vi "Main.vi"(8 "error in":errorcluster, 11 "Aging View in":refnum<class "Aging View.lvclass">) -> (0 "error out":errorcluster, 3 "Aging View out":refnum<class "Aging View.lvclass">)   [LabVIEW 2018, in "Aging View.lvclass"]
doc: "The Queued Message Handler of a Worker."
uses:
  Aging View.lvclass
  D:/Program Files (x86)/National Instruments/LabVIEW 2018/vi.lib/addons/_Workers/Library/Classes/Worker/Worker.lvclass
  Slot.ctl
  Initialization Data.ctl
  <vilib>/addons/_Workers/Library/Classes/Message Queue/Message Queue.lvclass
  Aging View.lvclass/Aging View.ctl
  <vilib>/addons/_Workers/Library/Classes/Message/Priority.ctl
  Datas.ctl
  <vilib>/addons/_Workers/Library/Classes/Message/Enqueue Message to Queue.vi
  <vilib>/addons/_Workers/Library/Classes/Message/Enqueue Message to Self v2.vi
  <vilib>/addons/_Workers/Library/Classes/Worker/Worker.lvclass
  <vilib>/addons/_Workers/Library/Classes/Message/Message.lvclass
  Acquire Data/Acquire Data.lvclass
  D:/Program Files (x86)/National Instruments/LabVIEW 2018/vi.lib/addons/_Workers/Library/Classes/Workers Object/Workers Object.lvclass
panel:
  out "Slot10":T1 {"Volt" format="%.2f"; "Temperature" format="%.2f"; "Current" format="%.2f"}
  out "Slot9":T1 {"Volt" format="%.2f"; "Temperature" format="%.2f"; "Current" format="%.2f"}
  out "Slot8":T1 {"Volt" format="%.2f"; "Temperature" format="%.2f"; "Current" format="%.2f"}
  out "Slot7":T1 {"Volt" format="%.2f"; "Temperature" format="%.2f"; "Current" format="%.2f"}
  out "Slot6":T1 {"Volt" format="%.2f"; "Temperature" format="%.2f"; "Current" format="%.2f"}
  out "Slot5":T1 {"Volt" format="%.2f"; "Temperature" format="%.2f"; "Current" format="%.2f"}
  out "Slot4":T1 {"Volt" format="%.2f"; "Temperature" format="%.2f"; "Current" format="%.2f"}
  out "Slot3":T1 {"Volt" format="%.2f"; "Temperature" format="%.2f"; "Current" format="%.2f"}
  out "Slot2":T1 {"Volt" format="%.2f"; "Temperature" format="%.2f"; "Current" format="%.2f"}
  out "Slot1":T1 {"Volt" format="%.2f"; "Temperature" format="%.2f"; "Current" format="%.2f"}
  in  "Stop Button":bool
  in  "Start Button":bool
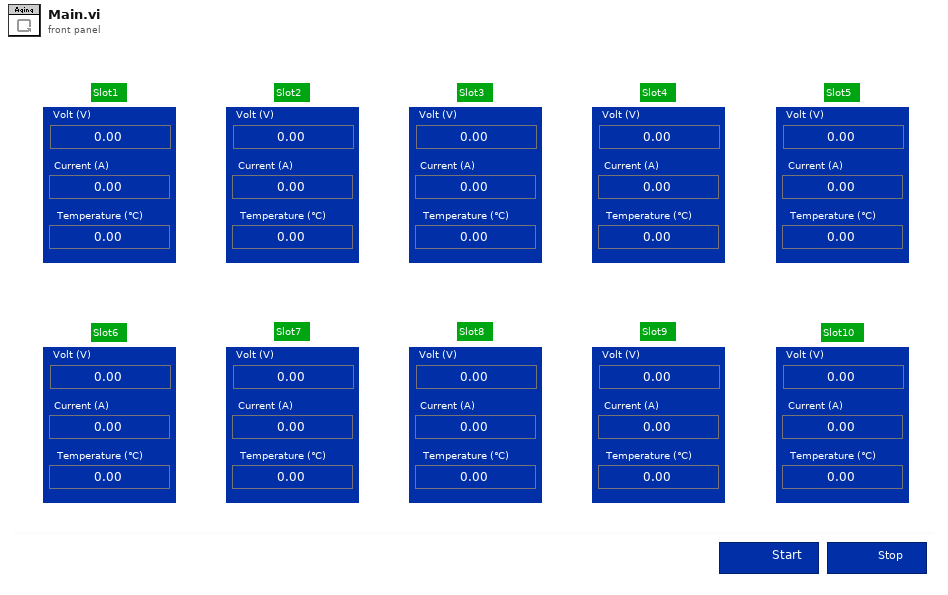
[diagram p1: front panel]
types:
  T1 = typedef "Aging View.lvclass/Slot.ctl" = cluster{"Current":dbl, "Temperature":dbl, "Volt":dbl}
  T2 = typedef "Aging View.lvclass/Initialization Data.ctl" = cluster{"MainPanel":refnum<vi>, "Acquire Queue":refnum<class "Message Queue.lvclass">}
  T3 = typedef "Workers.lvlib/Message.lvclass/Priority.ctl" = enum16{"Low", "Normal", "High"}
  T4 = typedef "Aging View.lvclass/Datas.ctl" = cluster{"Volts":dbl[], "Currents":dbl[], "Temps":dbl[]}
  T5 = typedef "Workers.lvlib/Case Label.ctl" = string
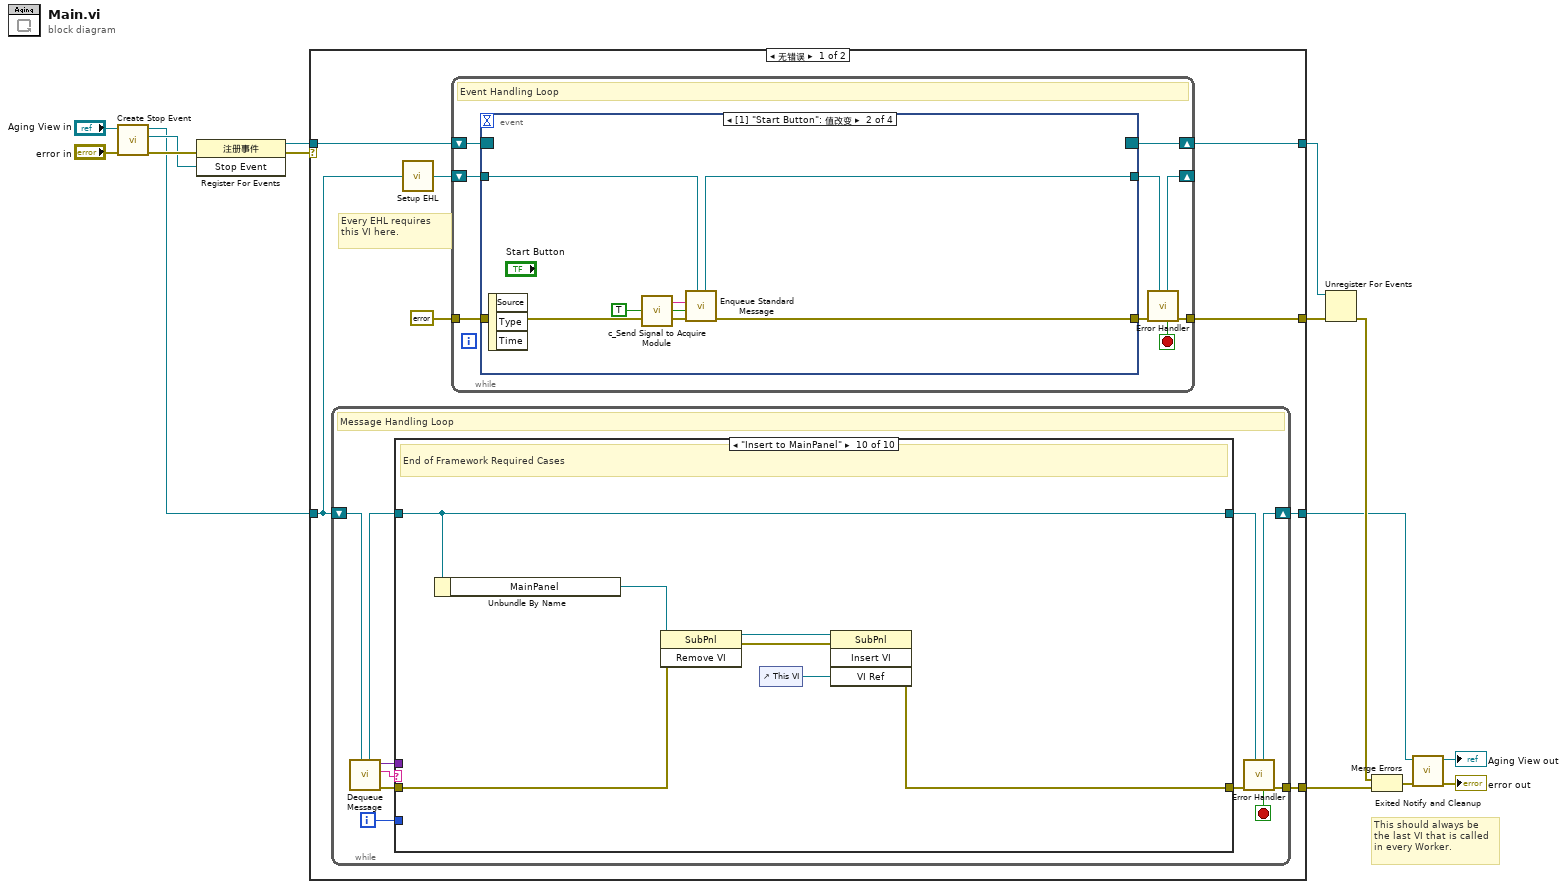
[diagram p0: block diagram]
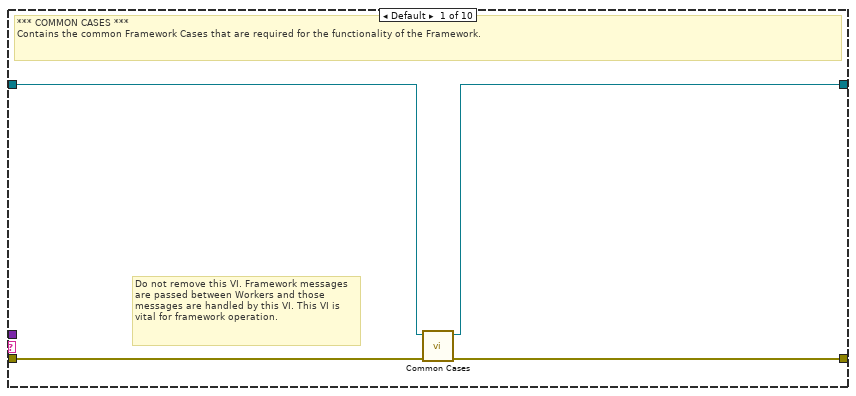
[diagram p2: hidden frame]
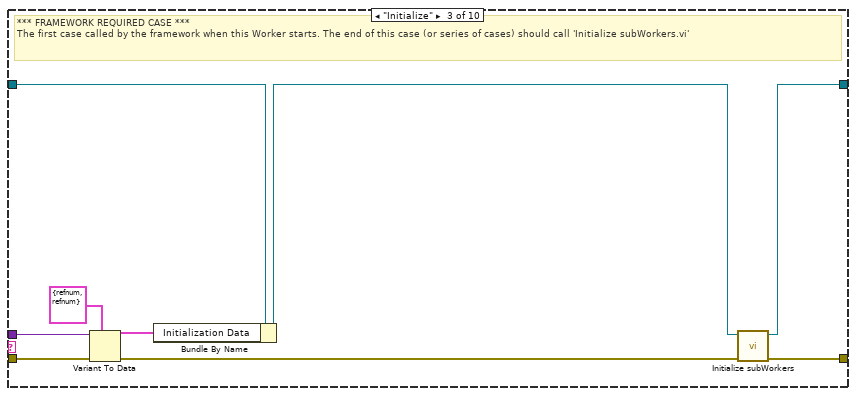
[diagram p4: hidden frame]
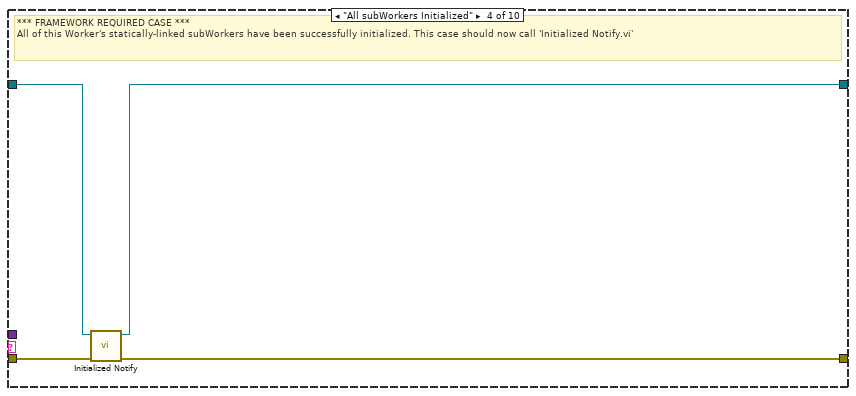
[diagram p5: hidden frame]
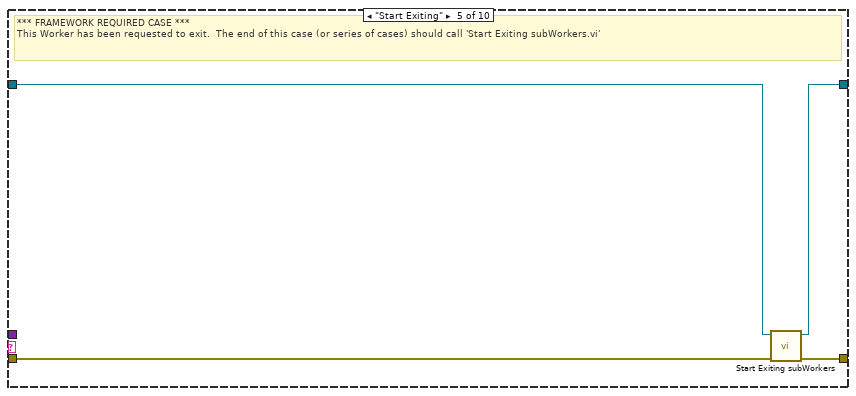
[diagram p6: hidden frame]
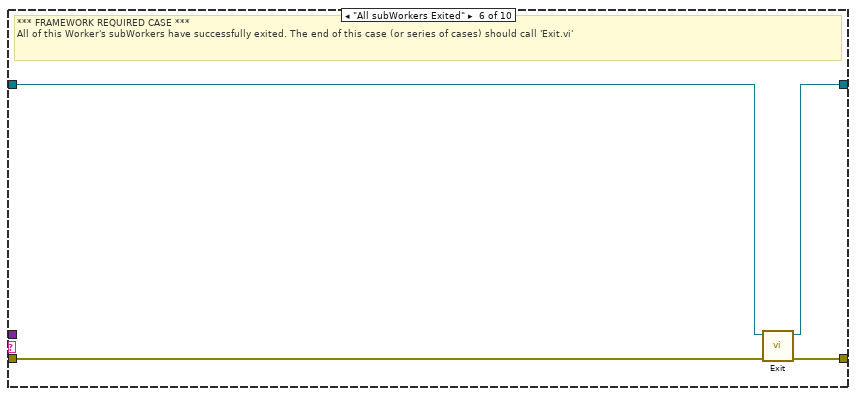
[diagram p7: hidden frame]
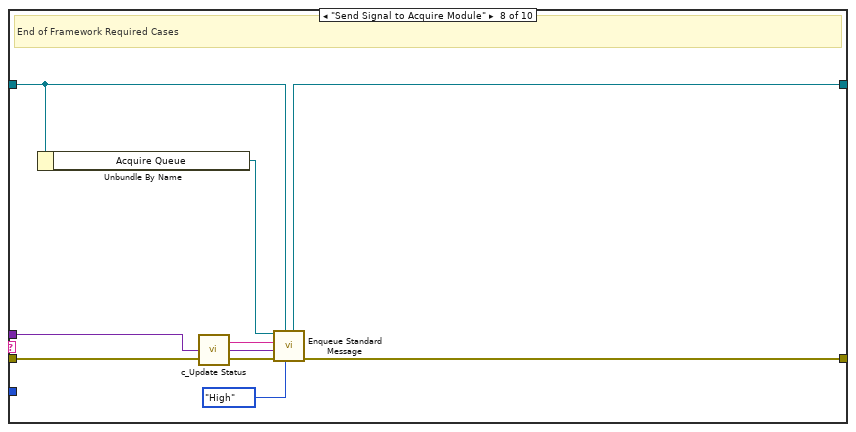
[diagram p9: hidden frame]
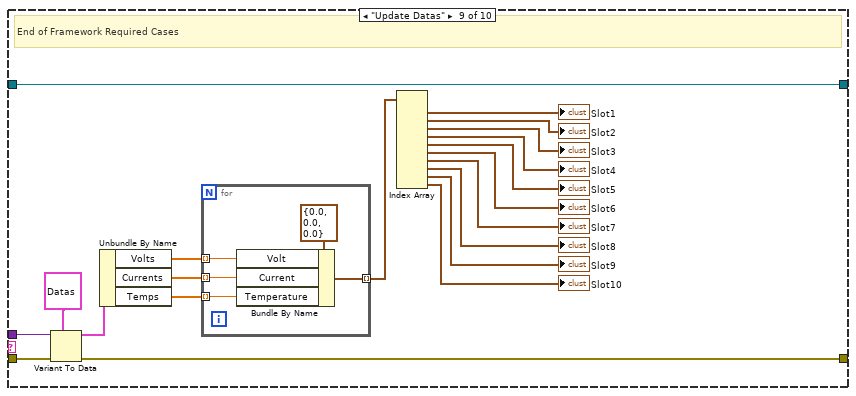
[diagram p10: hidden frame]
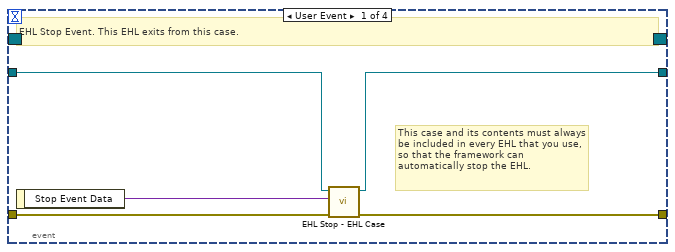
[diagram p11: hidden frame]
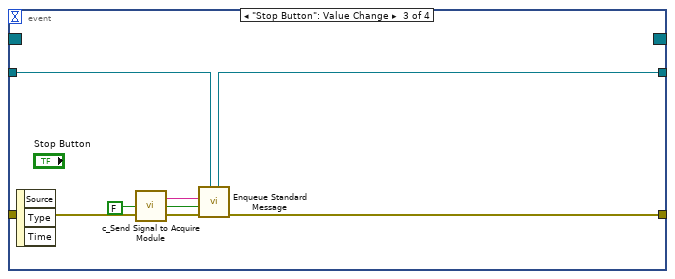
[diagram p12: hidden frame]
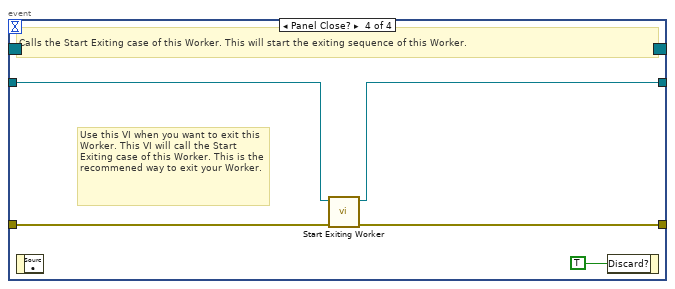
[diagram p13: hidden frame]
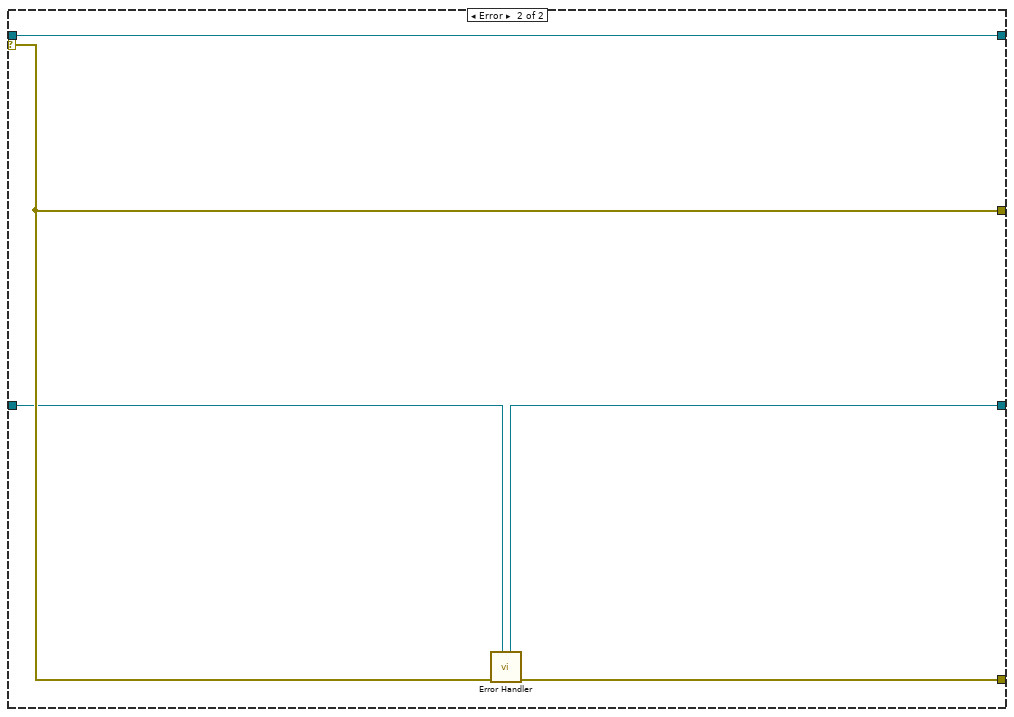
[diagram p14: hidden frame]
diagram:
  # "This should always be the last VI that is called in every Worker."
  n1 = call-dynamic "Create Stop Event.vi"("error in"="error in", "Worker"="Aging View in") -> ("error out"=w10:errorcluster, "Stop Event"=w7:refnum<user-event>, "Worker out"=w4:refnum<class "Aging View.lvclass">)  [unwired: 7 in]
  n2 = register-events(error in=w10, w7) -> (reference out=w9:refnum<event-registration>, error out=w1:errorcluster)  [unwired: 1 in]
  n3 = case shown="无错误" w1 {
    tunnel: w4 -> [w18 w136]
    tunnel: [w16 w137] -> w8
    tunnel: w9 -> [w23 w138]
    tunnel: [w20 w139] -> w14
    tunnel: [w22 w138] -> w13
    tunnel: [w17 w135] -> w11
    selector: w1 -> [_ w139]
    frame No Error {
      # "Every EHL requires\nthis VI here."
      n4 = while {
        shift-right: [w32] -> w17
        shift-left: w18 -> [w34]
        tunnel: [w33] -> w16
        i -> [w24]
        stop <- w25 stop-if-true
        # "Message Handling Loop"
        n5 = call-dynamic "Dequeue Message.vi"("Worker"=w34) -> ("error out"=w31:errorcluster, "Case out"=w26:string, "Data out"=w27:variant, "Worker out"=w29:refnum<class "Aging View.lvclass">)  [unwired: 6 in, 1 out]
        n6 = case "Worker MHL Case Structure (DO NOT CHANGE LABEL NAME)" shown="\"Insert to MainPanel\"" w26 {
          tunnel: w31 -> [w38 w39 w47 w51 w54 w61 w62 w70 w90 w99]
          tunnel: [w37 w39 w49 w50 w57 w60 w62 w71 w74 w98] -> w30
          tunnel: w29 -> [w36 w40 w43 w53 w55 w59 w63 w68 w75 w103]
          tunnel: [w35 w40 w48 w52 w56 w58 w63 w69 w75 w103] -> w28
          tunnel: w27 -> [_ _ w45 _ _ _ _ w65 w91 _]
          tunnel: w24 -> [_ _ _ _ _ _ _ _ _ _]
          frame Default {
            # "Do not remove this VI. Framework messages are passed between Workers and those messages are handled by this VI. This VI is vital for framework operation."
            # "*** COMMON CASES ***\nContains the common Framework Cases that are required for the functionality of the Framework."
            n7 = call-dynamic "Common Cases.vi"("error in"=w38, "Worker in"=w36) -> ("error out"=w37:errorcluster, "Worker out"=w35:refnum<class "Aging View.lvclass">)  [unwired: 8 in]
          }
          frame "------ FRAMEWORK REQUIRED CASES ------" {
            # "Start of Framework Required Cases"
          }
          frame "Initialize" {
            # "*** FRAMEWORK REQUIRED CASE ***\nThe first case called by the framework when this Worker starts. The end of this case (or series of cases) should call 'Initialize subWorkers.vi'"
            n8 = Variant To Data(error in=w47, type=T2 {"MainPanel"=refnum, "Acquire Queue"=refnum} ("Initialization Data"), Variant=w45) -> (data=w41:T2, error out=w46:errorcluster)
            n9 = Bundle By Name(cluster=w43, "Initialization Data"=w41) -> (w42:refnum<class "Aging View.lvclass">)
            n10 = call-dynamic "Initialize subWorkers.vi"("error in"=w46, "Worker"=w42) -> ("error out"=w49:errorcluster, "dup Worker out"=w48:refnum<class "Aging View.lvclass">)  [unwired: 8 in]
          }
          frame "All subWorkers Initialized" {
            # "*** FRAMEWORK REQUIRED CASE ***\nAll of this Worker's statically-linked subWorkers have been successfully initialized. This case should now call 'Initialized Notify.vi'"
            n11 = call-dynamic "Initialized Notify.vi"("error in"=w51, "Worker"=w53) -> ("error out"=w50:errorcluster, "dup Worker out"=w52:refnum<class "Aging View.lvclass">)  [unwired: 8 in]
          }
          frame "Start Exiting" {
            # "*** FRAMEWORK REQUIRED CASE ***\nThis Worker has been requested to exit.  The end of this case (or series of cases) should call 'Start Exiting subWorkers.vi'"
            n12 = call-dynamic "Start Exiting subWorkers.vi"("error_in"=w54, "Worker"=w55) -> ("error out"=w57:errorcluster, "dup Worker out"=w56:refnum<class "Aging View.lvclass">)  [unwired: 8 in]
          }
          frame "All subWorkers Exited" {
            # "*** FRAMEWORK REQUIRED CASE ***\nAll of this Worker's subWorkers have successfully exited. The end of this case (or series of cases) should call 'Exit.vi'"
            n13 = call-dynamic "Exit.vi"("error_in"=w61, "Worker"=w59) -> ("error out"=w60:errorcluster, "dup Worker out"=w58:refnum<class "Aging View.lvclass">)  [unwired: 8 in]
          }
          frame "-----------------------------------------------" {
            # "End of Framework Required Cases"
          }
          frame "Send Signal to Acquire Module" {
            # "End of Framework Required Cases"
            n14 = Unbundle By Name(w68) -> ("Acquire Queue"=w67:refnum<class "Message Queue.lvclass">)
            n15 = call "c_Update Status.vi"() -> ("Case Label"=w66:T5)  [unwired: 1 in]
            n16 = call-poly <vilib>:"Enqueue Standard Message.vi"("Priority (Normal)"=Priority."High", "Worker"=w68, "error in"=w70, "Data"=w65, "Case Label"=w66, "Message Queue"=w67) -> ("error out"=w71:errorcluster, "dup Worker out"=w69:refnum<class "Aging View.lvclass">)  [unwired: 3 in, 1 out]
          }
          frame "Update Datas" {
            # "End of Framework Required Cases"
            n17 = Variant To Data(error in=w90, type=T4 {"Volts"=[150.16634874669379, 153.68599144269746, 145.2965279660825, 150.72723584964493, 145.24862342605675, 148.81855123547712, 154.16505532014958, 149.4503630674569, 148.93848269644124, 147.4896592075], "Currents"=[150.16634874669379, 153.68599144269746, 145.2965279660825, 150.72723584964493, 145.24862342605675, 148.81855123547712, 154.16505532014958, 149.4503630674569, 148.93848269644124, 147.4896592075], "Temps"=[150.16634874669379, 153.68599144269746, 145.2965279660825, 150.72723584964493, 145.24862342605675, 148.81855123547712, 154.16505532014958, 149.4503630674569, 148.93848269644124, 147.4896592075]} ("Datas"), Variant=w91) -> (data=w88:T4, error out=w74:errorcluster)
            n18 = Unbundle By Name(w88) -> ("Volts"=w87:dbl[], "Currents"=w73:dbl[], "Temps"=w72:dbl[])
            n19 = for {
              tunnel: w87 -> [w95] mode=indexing
              tunnel: w73 -> [w94] mode=indexing
              tunnel: w72 -> [w93] mode=indexing
              tunnel: [w92] -> w86 mode=indexing
              n20 = Bundle By Name(cluster=T1 {"Current"=0.0, "Temperature"=0.0, "Volt"=0.0} ("Slot10"), "Volt"=w95, "Current"=w94, "Temperature"=w93) -> (w92:T1)
            }
            n21 = Index Array(array=w86) -> (element #1=→"Slot1":T1, element #2=→"Slot2":T1, element #3=→"Slot3":T1, element #4=→"Slot4":T1, element #5=→"Slot5":T1, element #6=→"Slot6":T1, element #7=→"Slot7":T1, element #8=→"Slot8":T1, element #9=→"Slot9":T1, element #10=→"Slot10":T1)  [unwired: 10 in]
          }
          frame "Insert to MainPanel" {
            # "End of Framework Required Cases"
            n22 = Unbundle By Name(w103) -> ("MainPanel"=w102:refnum<vi>)
            n23 = invoke class="SubPnl" method="Remove VI"(reference=w102, error in=w99) -> (reference out=w101:refnum<vi>, error out=w100:errorcluster)  [unwired: 1 in, 1 out]
            n24 = control-ref of="This VI"() -> (w97:refnum<vi>)
            n25 = invoke class="SubPnl" method="Insert VI"(reference=w101, error in=w100, "VI Ref"=w97) -> (error out=w98:errorcluster)  [unwired: 1 in, 3 out]
          }
        }
        n26 = call-dynamic "Error Handler.vi"("Worker"=w28, "error_in"=w30) -> ("error out"=w33:errorcluster, "Stop Loop"=w25:bool, "Worker out"=w32:refnum<class "Aging View.lvclass">)  [unwired: 7 in]
      }
      n27 = call-dynamic "Setup EHL.vi"("Worker"=w18) -> ("Worker out"=w19:refnum<class "Aging View.lvclass">)  [unwired: 14 in]
      n28 = while "Event Handling Loop" {
        shift-right: [w112] -> w22
        shift-left: w23 -> [w111]
        tunnel: [w107] -> w20
        tunnel: errorcluster {"status"=FALSE, "code"=0, "source"=""} ("error constant") -> [w109]
        shift-right: [w105] -> _
        shift-left: w19 -> [w110]
        stop <- w104 stop-if-true
        # "Event Handling Loop"
        n29 = event shown="[1] \"Start Button\": 值改变" {
          selector: w111 -> [_ _ _ _]
          dyn-events: [_ _ _ _] -> w112
          timeout: _ -> [_ _ _ _]
          tunnel: [w116 w122 w128 w133] -> w108
          tunnel: w109 -> [w117 w123 w129 w132]
          tunnel: w110 -> [w115 w120 w126 w131]
          tunnel: [w114 w121 w127 w130] -> w106
          event User Event {
            # "This case and its contents must always be included in every EHL that you use, so that the framework can automatically stop the EHL."
            # "EHL Stop Event. This EHL exits from this case."
            n30 = event-data() -> ("Stop Event Data"=w113:variant)  [unwired: 1 in]
            n31 = call <vilib>:"EHL Stop - EHL Case.vi"("error in"=w117, "Stop Event Data"=w113, "Worker"=w115) -> ("error out"=w116:errorcluster, "Worker out"=w114:refnum<class "Aging View.lvclass">)  [unwired: 7 in]
          }
          event "Start Button": Value Change {
            n32 = event-data() -> ()  [unwired: 1 in, 3 out]
            n33 = call "c_Send Signal to Acquire Module.vi"() -> ("Case Label"=w118:T5)  [unwired: 1 in]
            n34 = call-poly <vilib>:"Enqueue Standard Message.vi"("Worker"=w120, "error in"=w123, "Data"=TRUE, "Case Label"=w118) -> ("error out"=w122:errorcluster, "dup Worker out"=w121:refnum<class "Aging View.lvclass">)  [unwired: 6 in]
          }
          event "Stop Button": Value Change {
            n35 = event-data() -> ()  [unwired: 1 in, 3 out]
            n36 = call "c_Send Signal to Acquire Module.vi"() -> ("Case Label"=w124:T5)  [unwired: 1 in]
            n37 = call-poly <vilib>:"Enqueue Standard Message.vi"("Worker"=w126, "error in"=w129, "Data"=FALSE, "Case Label"=w124) -> ("error out"=w128:errorcluster, "dup Worker out"=w127:refnum<class "Aging View.lvclass">)  [unwired: 6 in]
          }
          event Panel Close? {
            # "Use this VI when you want to exit this Worker. This VI will call the Start Exiting case of this Worker. This is the recommened way to exit your Worker."
            # "Calls the Start Exiting case of this Worker. This will start the exiting sequence of this Worker."
            n38 = event-data() -> ()  [unwired: 1 in, 1 out]
            n39 = call-dynamic "Start Exiting Worker.vi"("error in"=w132, "Worker"=w131) -> ("error out"=w133:errorcluster, "dup Worker out"=w130:refnum<class "Aging View.lvclass">)  [unwired: 8 in]
            n40 = event-data("Discard?"=TRUE) -> ()  [unwired: 1 in, 1 out]
          }
        }
        n41 = call-dynamic "Error Handler.vi"("Worker"=w106, "error_in"=w108) -> ("error out"=w107:errorcluster, "Stop Loop"=w104:bool, "Worker out"=w105:refnum<class "Aging View.lvclass">)  [unwired: 7 in]
      }
    }
    frame Error {
      n42 = call-dynamic "Error Handler.vi"("Worker"=w136, "error_in"=w139) -> ("error out"=w137:errorcluster, "Worker out"=w135:refnum<class "Aging View.lvclass">)  [unwired: 7 in, 1 out]
    }
  }
  n43 = Unregister For Events(event registration refnum=w13, error in=w14) -> (error out=w15:errorcluster)
  n44 = Merge Errors(w15, w8) -> (w12:errorcluster)
  n45 = call-dynamic "Exited Notify and Cleanup.vi"("error_in"=w12, "Worker"=w11) -> ("error out"=→"error out":errorcluster, "dup Worker out"=→"Aging View out":refnum<class "Aging View.lvclass">)  [unwired: 8 in]
